vi "generate_calibration_lookup_2.3.vi"() -> ()   [LabVIEW 2019]
uses:
  2.3_subVIs/REFS.vi
panel:
  out "start (nearest)":dbl caption="Calibrated range"
  out "end (nearest)":dbl
  out "Zeroes":bool
  out "Phase":bool
  out "Read":bool
  in  "?":enum32{"Read", "Zeroes", "Phase", "Write"}(tab)
  out "Spectra folder error":errorcluster
  out "Voltage file error":errorcluster
  out "Zeroes outliers":dbl[](array[numeric])
  out "phase artifact wls":dbl[](array[numeric])
  in  "Phase warning":dbl=1.0
  out "Write error":errorcluster
  out "Write":bool
  out "Intensity Graph":dbl[][](graph)
  out "Saved":bool
  out "Task":string
  out "Task progress":u32(slide) scale=-1.1..640.0
  in  "Save":bool
  in  "Pixel":i32 min=1 max=640
  in  "Wavelength":dbl
  in  "Run":bool
  in  "stop":bool
  in  "Scrollbar V":i32(c297)
  in  "?":T1(tab)
  out "voltage-phase smoothed":T2(array[cluster])
  out "voltage-phase raw":T2(array[cluster])
  out "volt-amplitude":cluster{"XY Graph":cluster{"X":dbl[], dbl[]}}[](array[cluster])
  out "volt-offset":T2(array[cluster])
  in  "?":enum32{"File", "Pixel", "Bounds", "Processing"}(tab)
  in  "Spectra folder":path=path "C:/Users/User/Documents/2023S Peter/20230711/Master fixed, Slave scanned/Spectra folder"
  in  "Voltage file":path=path "C:/Users/User/Documents/2023S Peter/20230711/Master fixed, Slave scanned/Voltage folder/Voltage"
  in  "Calibration folder":path
  in  "Filename":string
  in  "Wavelengths":dbl[](array[numeric])=[812.46, 783.32]
  in  "Pixel numbers":i32[](array[numeric])=[146, 306]
  in  "Pixels":i32=640
  in  "Max":dbl=4095.0
  in  "Min":dbl=455.0
  in  "start":dbl=756.0 caption="Min"
  in  "end":dbl=816.0 caption="Max"
  in  "Window size":i32=11 min=0
  in  "xmin":dbl=600.0
  in  "Extrapolate":bool
  in  "xmax":dbl=2800.0
  out "voltage-transmission":T3(array[cluster])
  out "File location":path
  # "--"
  # "(nm)"
  # "VIEW"
  # "STATUS"
  # "Raw Transmission"
  # "Error code d7 means that the selected file/folder does not exist.\n\nSee online LabView documentation on \"Read Delimited Spreadsheet.vi\" error codes for other error details."
  # "The number of voltage-phase zeroes found at the following wavelengths are not the same as the expected number."
  # "The voltage-phase curves at the following wavelengths have (approx.) second derivative above the warning threshold. This may be due to an error in finding maxima or too much noise in the data."
  # "Use the control below to set the warning threshold to a different value."
  # "Warning threshold"
  # "See online LabView documentation on \"Write Delimited Spreadsheet.vi\" error codes for error details."
  # "IMPORT"
  # "EXPORT"
  # "CALIBRATION"
  # "SLM INFO"
  # "(nm)"
  # "VOLTAGE"
  # "WAVELENGTH"
  # "(counts)"
  # "(counts)"
  # "(nm)"
  # "(nm)"
  # "DENOISING"
  # "ZEROES"
  # "ERROR CORRECTION"
  # "Find between"
  # "(counts)"
  # "(counts)"
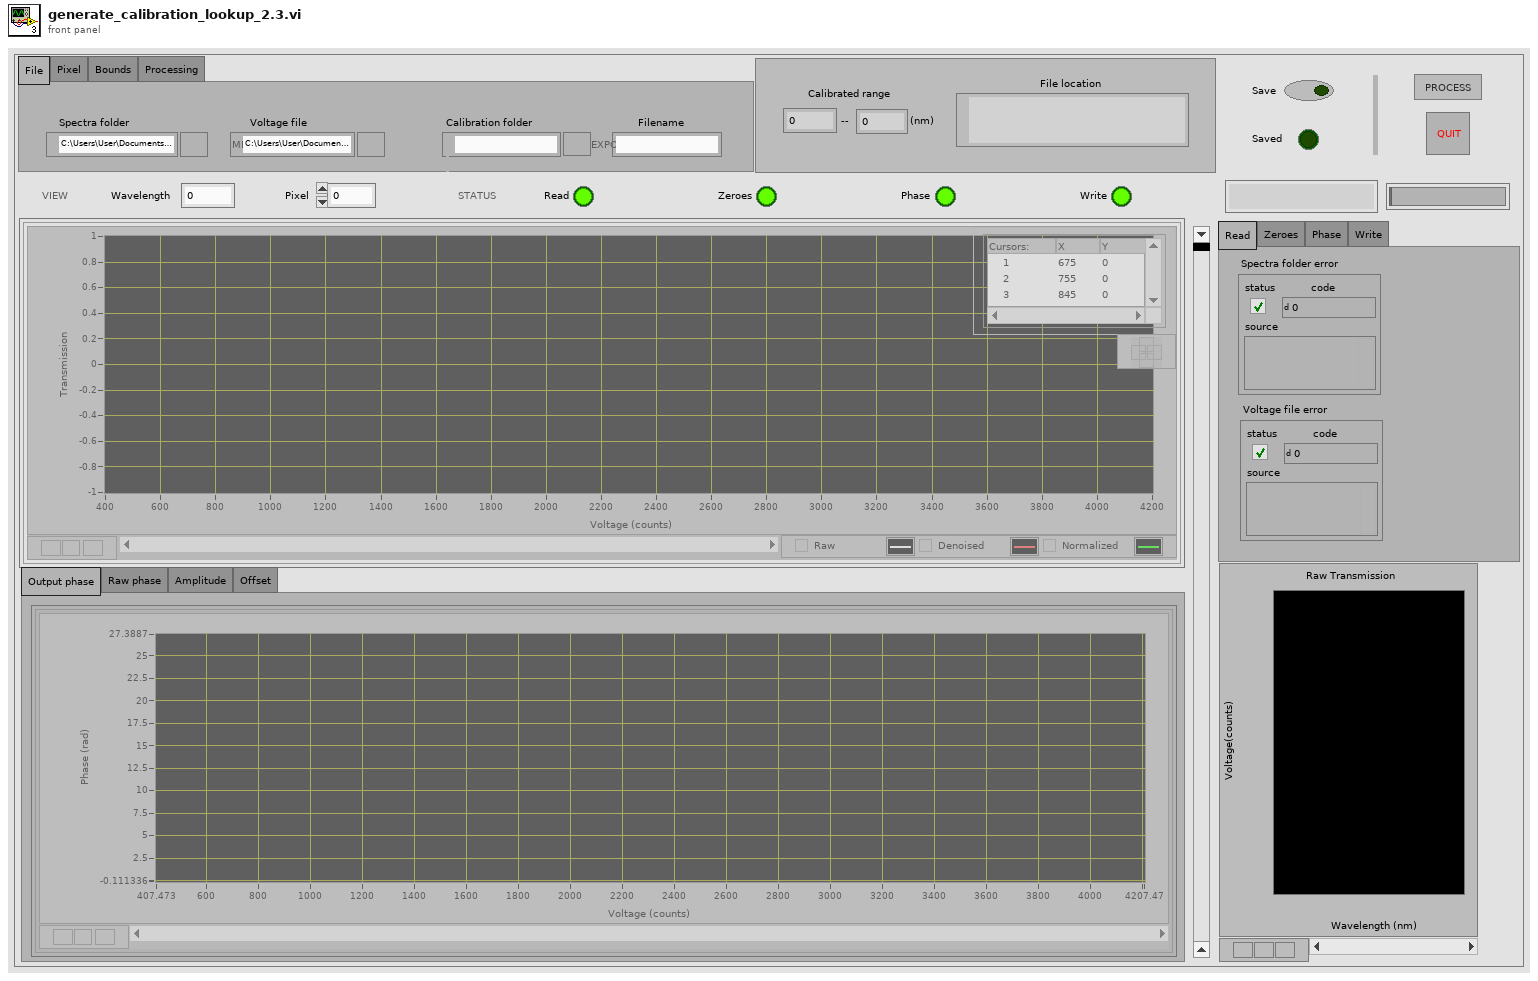
[diagram p1: front panel]
types:
  T1 = enum32{"Output phase", "Raw phase", "Amplitude", "Offset"}
  T2 = cluster{"XY Graph":cluster{"X":dbl[], "Phase":dbl[]}}[]
  T3 = cluster{"XY Graph":cluster{"X":dbl[], "Transmission":dbl[]}[]}[]
  T4 = cluster{"Extrema (type, idx)":cluster{"extrema type":bool, i32}[]}[]
  T5 = cluster{"trunc voltages":dbl[], "transmissions[r=wl, c=v]":dbl[]}
  T6 = cluster{"remaining volts":dbl[], "smoothed transmissions[r=wl,c=v]":dbl[]}
  T7 = cluster{"Voltages out":dbl[], "Locally normalized transmission (r=wl, c=v)":dbl[]}
  T8 = cluster{"Voltages out":dbl[], "Locally normalized transmission (r=wl, c=v)":dbl[]}[]
  T9 = cluster{cluster{"Voltages out":dbl[], "Locally normalized transmission (r=wl, c=v)":dbl[]}[]}
  T10 = cluster{"Zeroes":bool, "Phase":bool, "Zeroes outliers":dbl[], "phase artifact wls":dbl[]}
  T11 = cluster{"Voltages out":dbl[], "Phase (r=wl, c=v)":dbl[]}
  T12 = cluster{"Voltages out":dbl[], "Phase out (r=wl, c=v)":dbl[]}
  T13 = cluster{cluster{"Voltages out":dbl[], "Phase (r=wl, c=v)":dbl[]}}
  T14 = cluster{cluster{"Voltages out":dbl[], "Phase out (r=wl, c=v)":dbl[]}}
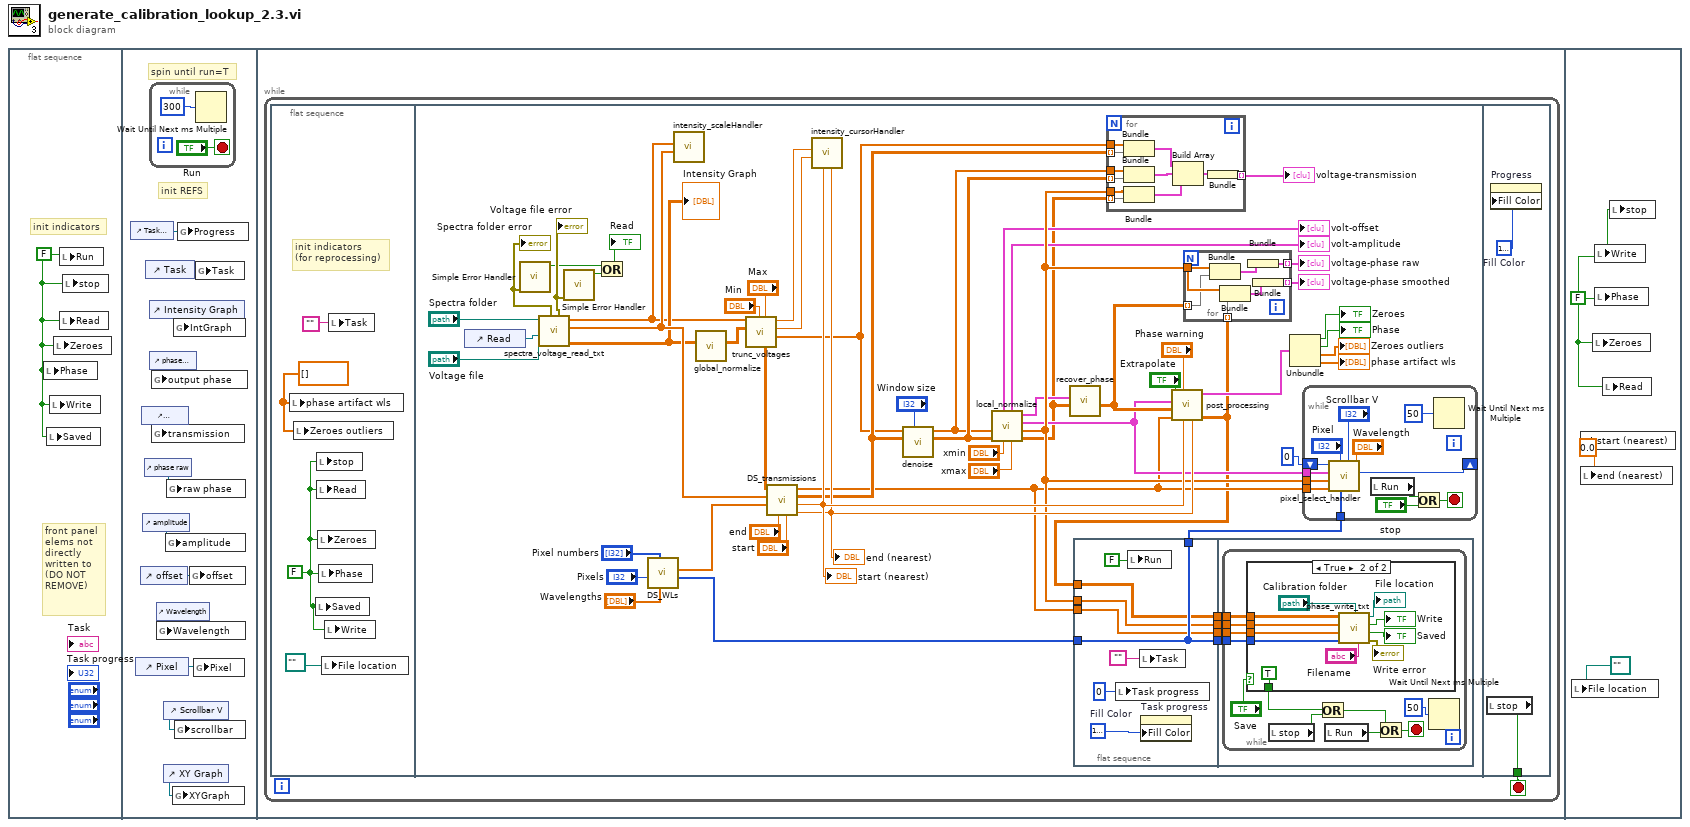
[diagram p0: block diagram]
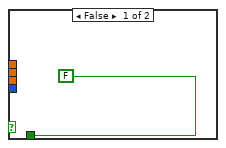
[diagram p2: hidden frame]
diagram:
  n1 = flat-sequence {
    frame #0 {
      w1 = FALSE
      # "init indicators"
      # "front panel elems not directly written to (DO NOT REMOVE)"
      n2 = local write "Phase"(w1) -> ()
      n3 = local write "Saved"(w1) -> ()
      n4 = local write "Write"(w1) -> ()
      n5 = local write "Zeroes"(w1) -> ()
      n6 = local write "Run"(w1) -> ()
      n7 = local write "Read"(w1) -> ()
      n8 = local write "stop"(w1) -> ()
    }
    frame #1 {
      # "init REFS"
      # "spin until run=T"
      n9 = control-ref of="Task progress"() -> (w12:refnum<vi>)
      n10 = control-ref of="Pixel"() -> (w8:refnum<vi>)
      n11 = control-ref of="offset"() -> (w6:refnum<vi>)
      n12 = control-ref of="transmission"() -> (w3:refnum<vi>)
      n13 = control-ref of="amplitude"() -> (w5:refnum<vi>)
      n14 = control-ref of="phase raw"() -> (w4:refnum<vi>)
      n15 = control-ref of="Task"() -> (w11:refnum<vi>)
      n16 = while {
        stop <- "Run" stop-if-true
        n17 = Wait Until Next ms Multiple(millisecond multiple=300) -> ()  [unwired: 1 out]
      }
      n18 = control-ref of="Intensity Graph"() -> (w13:refnum<vi>)
      n19 = control-ref of="phase output"() -> (w2:refnum<vi>)
      n20 = global write "REFS.vi" "output phase"(w2) -> ()
      n21 = global write "REFS.vi" "transmission"(w3) -> ()
      n22 = control-ref of="Wavelength"() -> (w7:refnum<vi>)
      n23 = global write "REFS.vi" "Wavelength"(w7) -> ()
      n24 = control-ref of="Scrollbar V"() -> (w9:refnum<vi>)
      n25 = control-ref of="XY Graph"() -> (w10:refnum<vi>)
      n26 = global write "REFS.vi" "amplitude"(w5) -> ()
      n27 = global write "REFS.vi" "raw phase"(w4) -> ()
      n28 = global write "REFS.vi" "XYGraph"(w10) -> ()
      n29 = global write "REFS.vi" "IntGraph"(w13) -> ()
      n30 = global write "REFS.vi" "scrollbar"(w9) -> ()
      n31 = global write "REFS.vi" "Progress"(w12) -> ()
      n32 = global write "REFS.vi" "offset"(w6) -> ()
      n33 = global write "REFS.vi" "Pixel"(w8) -> ()
      n34 = global write "REFS.vi" "Task"(w11) -> ()
    }
    frame #2 {
      n35 = while {
        stop <- w16 stop-if-true
        n36 = flat-sequence {
          tunnel: [w145] -> w16
          frame #0 {
            w20 = dbl[] []
            w18 = FALSE
            # "init indicators\n(for reprocessing)"
            n37 = local write "phase artifact wls"(w20) -> ()
            n38 = local write "Zeroes outliers"(w20) -> ()
            n39 = local write "Saved"(w18) -> ()
            n40 = local write "stop"(w18) -> ()
            n41 = local write "Read"(w18) -> ()
            n42 = local write "Zeroes"(w18) -> ()
            n43 = local write "Phase"(w18) -> ()
            n44 = local write "File location"(path "" ("File location")) -> ()
            n45 = local write "Write"(w18) -> ()
            n46 = local write "Task"("") -> ()
          }
          frame #1 {
            n47 = control-ref of="Read"() -> (w23:refnum<vi>)
            n48 = call "spectra_voltage_read_txt.vi"("VOLTAGE_PATH"="Voltage file", "Boolean ref in"=w23, "SPECTRA_DIRECTORY"="Spectra folder") -> ("transmissions[r=wl, c=v]"=w77:dbl[][], "wavelengths"=w78:dbl[], "voltages"=w38:dbl[], "voltage file errors"=w27:errorcluster, "spectra directory errors"=w28:errorcluster)  [unwired: 4 in]
            "Intensity Graph" <- w77
            "Spectra folder error" <- w28
            "Voltage file error" <- w27
            n49 = call <vilib>:"Simple Error Handler.vi"("error in (no error)"=w28) -> ("error?"=w26:bool)  [unwired: 4 in, 4 out]
            n50 = call <vilib>:"Simple Error Handler.vi"("error in (no error)"=w27) -> ("error?"=w25:bool)  [unwired: 4 in, 4 out]
            n51 = Or(x=w26, y=w25) -> (x .or. y?=→"Read":bool)
            n52 = call "DS_WLs.vi"("Wavelengths"="Wavelengths", "Pixel numbers"="Pixel numbers", "Pixels"="Pixels") -> ("Pixels"=w36:i32[], "DSd WLs"=w59:dbl[])  [unwired: 7 in]
            n53 = call "intensity_scaleHandler.vi"("wavelengths"=w78, "voltages"=w38) -> ()  [unwired: 10 in]
            n54 = call "global_normalize.vi"("trunc_transmission[r=wl, c=v]"=w77) -> ("normalized transmission[r=wl, c=v]"=w53:dbl[][])  [unwired: 10 in]
            n55 = call "trunc_voltages.vi"("Max"="Max", "Min"="Min", "transmissions[r=wl, c=v]"=w53, "voltages"=w38) -> ("trunc voltages"=w42:dbl[], "Min"=w69:dbl, "Max"=w70:dbl, "trunc transmissions[r=wl, c=v]"=w43:dbl[][])  [unwired: 4 in]
            n56 = call "DS_transmissions.vi"("start"="start", "end"="end", "xi in"=w59, "wavelengths"=w78, "trunc transmissions[r=wl, c=v]"=w43) -> ("end (out)"=w75:dbl, "start (out)"=w76:dbl, "transmissions[r=wl, c=v]"=w73:dbl[][], "xi used"=w32:dbl[])  [unwired: 3 in]
            "end (nearest)" <- w75
            "start (nearest)" <- w76
            n57 = call "intensity_cursorHandler.vi"("End"=w75, "Start"=w76, "Min"=w69, "Max"=w70) -> ()  [unwired: 8 in]
            n58 = call "denoise.vi"("Window size"="Window size", "transmissions[r=wl,c=v]"=w73, "voltages"=w42) -> ("smoothed transmissions[r=wl,c=v]"=w52:dbl[][], "remaining volts"=w51:dbl[])  [unwired: 7 in]
            n59 = call "local_normalize.vi"("xmax"="xmax", "xmin"="xmin", "denoised transmission[r=wl, c=v]"=w52, "voltages in"=w51) -> ("Locally normalized transmission (r=wl, c=v)"=w21:dbl[][], "Voltages out"=w74:dbl[], "Zeroes (idx)"=w40:cluster{"Splice indices":i32[]}[], "Extrema (type, idx)"=w64:T4, "amplitude graphs"=→"volt-amplitude":cluster{"Amplitude":cluster{"X":dbl[], dbl[]}}[], "offset graphs"=→"volt-offset":cluster{"Offset":cluster{"X":dbl[], dbl[]}}[])  [unwired: 2 in]
            n60 = call "recover_phase.vi"("Normalized transmission (r=wl, c=v)"=w21, "Extrema (type, idx)"=w64) -> ("Phase (r=wl, c=v)"=w47:dbl[][])  [unwired: 9 in]
            n61 = flat-sequence {
              tunnel: [w113] -> w72
              tunnel: w74 -> [w113]
              tunnel: [w110] -> w71
              tunnel: w32 -> [w111]
              tunnel: [w111] -> w49
              tunnel: w36 -> [w117]
              tunnel: [w117] -> w37
              tunnel: w31 -> [w110]
              tunnel: [w117] -> w30
              tunnel: w72 -> [w121]
              tunnel: w71 -> [w118]
              tunnel: w49 -> [w120]
              tunnel: w37 -> [w119]
              frame #0 {
                w114 = u32 16777216  # Fill Color
                n62 = local write "Task progress"(u8 0 ("Task progress")) -> ()
                n63 = local write "Run"(FALSE) -> ()
                n64 = local write "Task"("") -> ()
                n65 = property on="Task progress" class="Slide (strict)"("Fill Color"=w114) -> ()  [unwired: 2 in, 2 out]
              }
              frame #1 {
                n66 = while {
                  tunnel: w120 -> [w130]
                  tunnel: w121 -> [w129]
                  tunnel: w119 -> [w123]
                  tunnel: w118 -> [w122]
                  stop <- w126 stop-if-true
                  n67 = case shown="True" "Save" {
                    tunnel: [FALSE TRUE] -> w128
                    tunnel: w130 -> [_ w137]
                    tunnel: w129 -> [_ w138]
                    tunnel: w123 -> [_ w135]
                    tunnel: w122 -> [_ w134]
                    frame False {
                    }
                    frame True {
                      n68 = call "phase_write_txt.vi"("Filename"="Filename", "Calibration folder"="Calibration folder", "pixels"=w135, "wavelengths"=w137, "voltages"=w138, "phase"=w134) -> ("error out"=→"Write error":errorcluster, "Boolean"=→"Saved":bool, "error?"=→"Write":bool, "new file path (Not A Path if cancelled)"=→"File location":path)  [unwired: 2 in]
                    }
                  }
                  n69 = local read "stop"() -> (w127:bool)
                  n70 = Or(x=w128, y=w127) -> (x .or. y?=w125:bool)
                  n71 = local read "Run"() -> (w124:bool)
                  n72 = Or(x=w125, y=w124) -> (x .or. y?=w126:bool)
                  n73 = Wait Until Next ms Multiple(millisecond multiple=u32 50) -> ()  [unwired: 1 out]
                }
              }
            }
            n74 = for {
              tunnel: w21 -> [w102] mode=indexing
              tunnel: w74 -> [w92]
              tunnel: [w99] -> w54 mode=indexing
              tunnel: w52 -> [w96] mode=indexing
              tunnel: w73 -> [w95] mode=indexing
              tunnel: w51 -> [w94]
              tunnel: w42 -> [w93]
              n75 = Bundle("trunc voltages"=w93, "transmissions[r=wl, c=v]"=w95) -> (w97:T5)  [unwired: 1 in]
              n76 = Bundle("remaining volts"=w94, "smoothed transmissions[r=wl,c=v]"=w96) -> (w98:T6)  [unwired: 1 in]
              n77 = Bundle("Voltages out"=w92, "Locally normalized transmission (r=wl, c=v)"=w102) -> (w100:T7)  [unwired: 1 in]
              n78 = Build Array(w97, w98, w100) -> (w101:T8)
              n79 = Bundle(w101) -> (w99:T9)  [unwired: 1 in]
            }
            "voltage-transmission" <- w54
            n80 = call "post_processing.vi"("wl end"=w75, "wl start"=w76, "Phase warning"="Phase warning", "Wavelengths"=w32, "Phase in (r=wl, c=v)"=w47, "Zeroes (idx)"=w40, "Extrapolate"="Extrapolate") -> ("Phase out (r=wl, c=v)"=w31:dbl[][], "Errors"=w62:T10)  [unwired: 3 in]
            n81 = for {
              tunnel: w74 -> [w104]
              tunnel: [w109] -> w56 mode=indexing
              tunnel: w31 -> [w107] mode=indexing
              tunnel: [w105] -> w55 mode=indexing
              tunnel: w47 -> [w103] mode=indexing
              n82 = Bundle("Voltages out"=w104, "Phase (r=wl, c=v)"=w103) -> (w108:T11)  [unwired: 1 in]
              n83 = Bundle("Voltages out"=w104, "Phase out (r=wl, c=v)"=w107) -> (w106:T12)  [unwired: 1 in]
              n84 = Bundle(w108) -> (w109:T13)  [unwired: 1 in]
              n85 = Bundle(w106) -> (w105:T14)  [unwired: 1 in]
            }
            "voltage-phase raw" <- w56
            "voltage-phase smoothed" <- w55
            n86 = Unbundle(w62) -> ("Zeroes"=→"Zeroes":bool, "Phase"=→"Phase":bool, "Zeroes outliers"=→"Zeroes outliers":dbl[], "phase artifact wls"=→"phase artifact wls":dbl[])
            n87 = while {
              tunnel: w32 -> [w90]
              shift-right: [w82] -> _
              shift-left: 0 -> [w83]
              tunnel: w40 -> [w85]
              tunnel: w74 -> [w84]
              tunnel: w30 -> [w80]
              stop <- w87 stop-if-true
              n88 = call "pixel_select_handler.vi"("Wavelength"="Wavelength", "Scrollbar V"="Scrollbar V", "Pixels"=w80, "Pixel"="Pixel", "Wavelengths"=w90, "Voltages"=w84, "Zeroes (idx)"=w85, "Curr idx"=w83) -> ("New idx"=w82:u32)  [unwired: 3 in]
              n89 = local read "Run"() -> (w86:bool)
              n90 = Or(x=w86, y="stop") -> (x .or. y?=w87:bool)
              n91 = Wait Until Next ms Multiple(millisecond multiple=u32 50) -> ()  [unwired: 1 out]
            }
          }
          frame #2 {
            w146 = u32 16777216  # Fill Color
            n92 = local read "stop"() -> (w145:bool)
            n93 = property on="Progress" class="Slide (strict)"("Fill Color"=w146) -> ()  [unwired: 2 in, 2 out]
          }
        }
      }
    }
    frame #3 {
      w148 = 0.0 ("start")
      w149 = FALSE
      n94 = local write "File location"(path "" ("File location")) -> ()
      n95 = local write "start (nearest)"(w148) -> ()
      n96 = local write "end (nearest)"(w148) -> ()
      n97 = local write "Zeroes"(w149) -> ()
      n98 = local write "Write"(w149) -> ()
      n99 = local write "Phase"(w149) -> ()
      n100 = local write "Read"(w149) -> ()
      n101 = local write "stop"(w149) -> ()
    }
  }
